vi "Button Sequencing.vi"(3 "2":bool, 6 "1":bool) -> (0 "Boolean":bool)   [LabVIEW 2019]
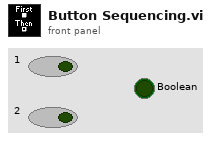
[diagram p1: front panel]
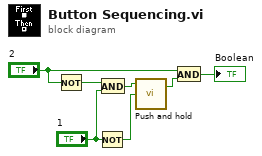
[diagram p0: block diagram]
diagram:
  n1 = Not(x="2") -> (.not. x?=w7:bool)
  n2 = Not(x="1") -> (.not. x?=w5:bool)
  n3 = And(x=w7, y="1") -> (x .and. y?=w6:bool)
  n4 = call "Push and hold.vi"("Reset"=w5, "Input"=w6) -> ("Output"=w3:bool)  [unwired: 2 in]
  n5 = And(x="2", y=w3) -> (x .and. y?=→"Boolean":bool)
